vi "Solve_Special_PRB_101_Subtracks-2.vi"(3 "error IN":errorcluster, 5 "[IN] Subtracks":T1(array[cluster])) -> (0 "error OUT":errorcluster, 1 "[OUT] Special case!":bool, 2 "[OUT] Subtracks":T1(array[cluster]))   [LabVIEW 2013]
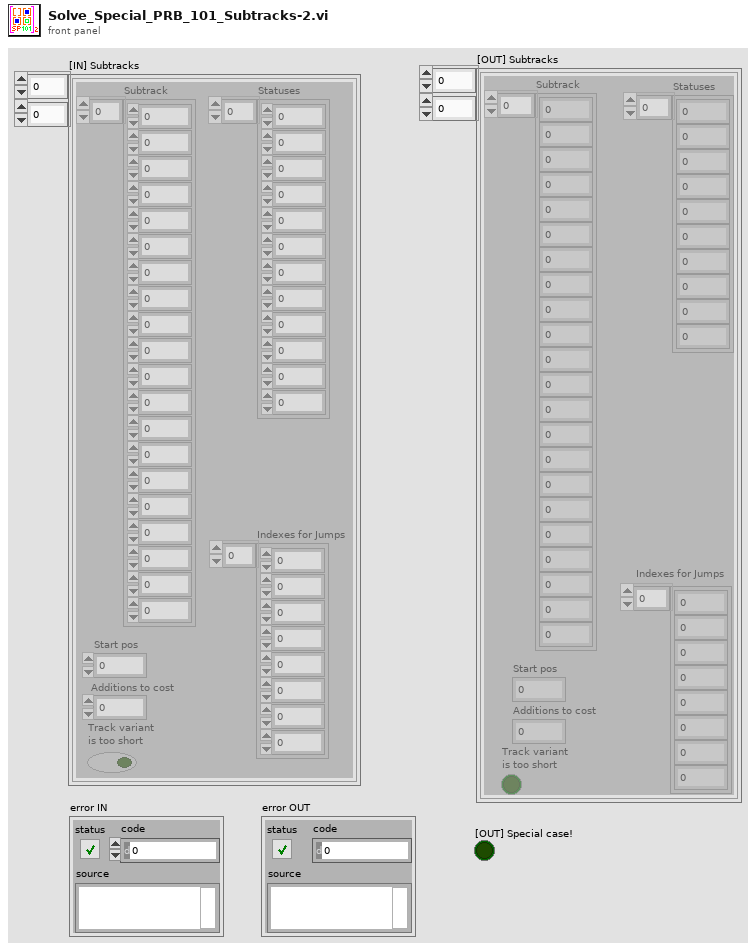
[diagram p1: front panel]
types:
  T1 = cluster{"Subtrack":dbl[], "Statuses":i16[], "Start pos":i32, "Additions to cost":i32, "Track variant \nis too short":bool, "Indexes for Jumps":i32[]}[][]
  T2 = cluster{"Subtrack":dbl[], "Statuses":i16[], "Start pos":i32, "Additions to cost":i32, "Track variant \nis too short":bool, "Indexes for Jumps":i32[]}
  T3 = cluster{"Subtrack":dbl[], "Statuses":i16[], "Start pos":i32, "Additions to cost":i32, "Track variant \nis too short":bool, "Indexes for Jumps":i32[]}[]
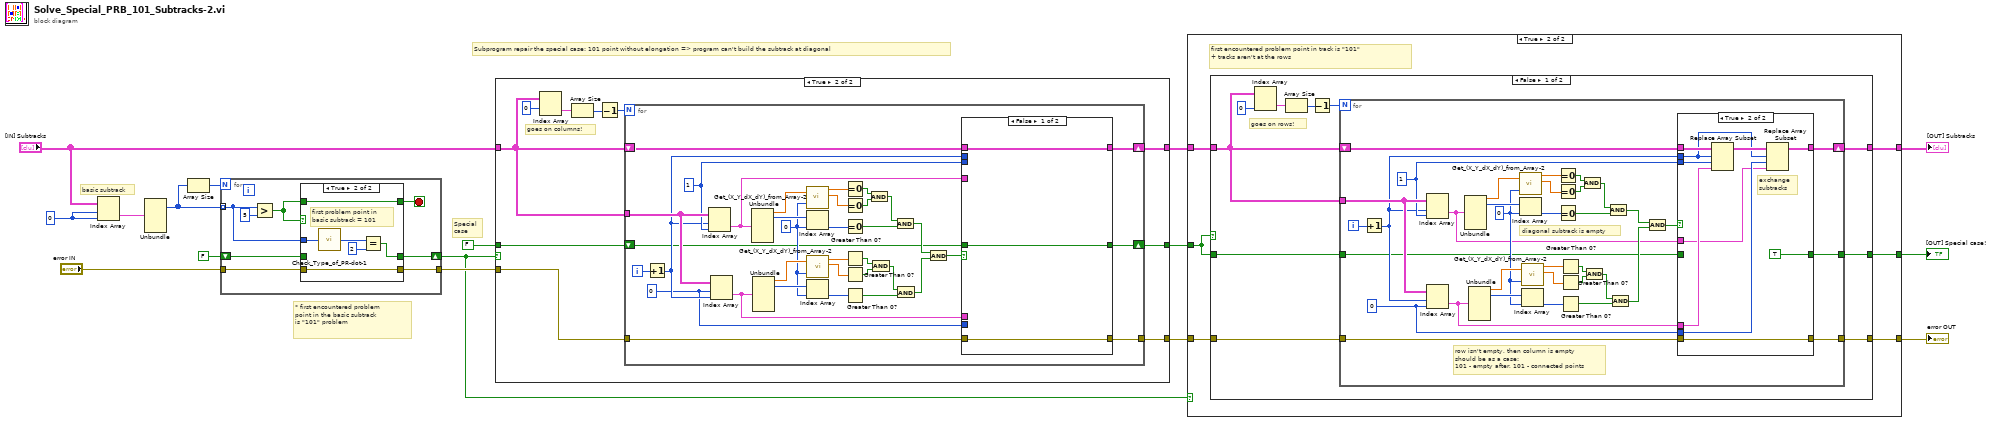
[diagram p0: block diagram]
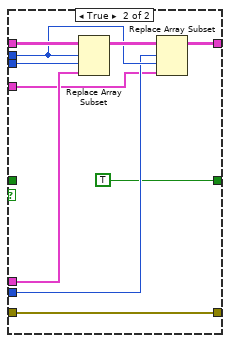
[diagram p6: hidden frame]
diagram:
  w16 = 0 ("index (row)")
  # "* first encountered problem\npoint in the basic subtrack\nis \"101\" problem"
  # "Special \ncase"
  # "Subprogram repair the special case: 101 point without elongation => program can't build the subtrack at diagonal"
  # "basic subtrack"
  n1 = Index Array(array="[IN] Subtracks", index (row)=w16, index (col)=w16) -> (element=w15:T2)
  n2 = Unbundle(w15) -> ("Statuses"=w13:i16[])  [unwired: 5 out]
  n3 = Array Size(array=w13) -> (size(s)=w14:i32)
  n4 = for {
    N: w14 -> [_]
    tunnel: w13 -> [w23] mode=indexing
    shift-right: [w19] -> w7
    shift-left: FALSE -> [w22]
    tunnel: "error IN" -> [w18]
    tunnel: [w17] -> w10
    stop <- w20 stop-if-true
    n5 = Greater?(x=w23, y=i16 5) -> (0:w21:bool)
    n6 = case shown="True" w21 {
      tunnel: w23 -> [_ w31]
      tunnel: w22 -> [w26 _]
      tunnel: w21 -> [w27 w30]
      tunnel: [w27 w30] -> w20
      tunnel: [w26 w29] -> w19
      tunnel: w18 -> [w25 w28]
      tunnel: [w25 w28] -> w17
      frame False {
      }
      frame True {
        # "first problem point in \nbasic subtrack = 101"
        n7 = call "Check_Type_of_PR-dot-1.vi"("[IN] dot status"=w31) -> ("[OUT] Type of\nproblem dot"=w33:i32)
        n8 = Equal?(x=w33, y=2) -> (x = y?=w29:bool)
      }
    }
  }
  n9 = case shown="True" w7 {
    tunnel: w10 -> [w35 w42]
    tunnel: "[IN] Subtracks" -> [w36 w45]
    tunnel: [w36 w40] -> w5
    tunnel: [w35 w41] -> w4
    tunnel: FALSE -> [w34 w39]
    tunnel: [w34 w38] -> w6
    frame False {
    }
    frame True {
      # "goes on columns!"
      n10 = Index Array(array=w45, index (row)=0 ("disabled index (col)")) -> (element=w46:T3)  [unwired: 1 in]
      n11 = Array Size(array=w46) -> (size(s)=w44:i32)
      n12 = Decrement(x=w44) -> (x-1=w43:i32)
      n13 = for {
        N: w43 -> [_]
        tunnel: w45 -> [w80]
        shift-right: [w51] -> w40
        shift-left: w45 -> [w57]
        tunnel: w42 -> [w50]
        tunnel: [w49] -> w41
        shift-right: [w47] -> w38
        shift-left: w39 -> [w48]
        i -> [w81]
        w65 = 0 ("index")
        w52 = 0 ("disabled index (col)")
        w54 = 1 ("disabled index (col)")
        n14 = Increment(x=w81) -> (x+1=w53:i32)
        n15 = Index Array(array=w80, index (row)=w53, index (col)=w54) -> (element=w56:T2)
        n16 = Index Array(array=w80, index (row)=w52, index (col)=w53) -> (element=w55:T2)
        n17 = Unbundle(w56) -> ("Subtrack"=w77:dbl[], "Statuses"=w79:i16[])  [unwired: 4 out]
        n18 = Unbundle(w55) -> ("Subtrack"=w76:dbl[], "Statuses"=w78:i16[])  [unwired: 4 out]
        n19 = call "Get_(X_Y_dX_dY)_from_Array-2.vi"("(X,Y,dX,dY)"=w77, "Index of Displacement"=w65) -> ("X"=w75:dbl, "Y"=w74:dbl)  [unwired: 2 out]
        n20 = Index Array(array=w79, index=w65) -> (element=w73:i16)
        n21 = call "Get_(X_Y_dX_dY)_from_Array-2.vi"("(X,Y,dX,dY)"=w76, "Index of Displacement"=w65) -> ("X"=w68:dbl, "Y"=w67:dbl)  [unwired: 2 out]
        n22 = Index Array(array=w78, index=w65) -> (element=w66:i16)
        n23 = Equal To 0?(x=w75) -> (x = 0?=w72:bool)
        n24 = Equal To 0?(x=w74) -> (x = 0?=w71:bool)
        n25 = Equal To 0?(x=w73) -> (x = 0?=w69:bool)
        n26 = Greater Than 0?(x=w68) -> (x > 0?=w64:bool)
        n27 = Greater Than 0?(x=w67) -> (x > 0?=w63:bool)
        n28 = Greater Than 0?(x=w66) -> (x > 0?=w61:bool)
        n29 = And(x=w72, y=w71) -> (x .and. y?=w70:bool)
        n30 = And(x=w64, y=w63) -> (x .and. y?=w62:bool)
        n31 = And(x=w70, y=w69) -> (x .and. y?=w60:bool)
        n32 = And(x=w62, y=w61) -> (x .and. y?=w59:bool)
        n33 = And(x=w60, y=w59) -> (x .and. y?=w58:bool)
        n34 = case shown="False" w58 {
          tunnel: w57 -> [w84 w94]
          tunnel: w56 -> [_ w88]
          tunnel: w55 -> [_ w92]
          tunnel: w53 -> [_ w90]
          tunnel: w54 -> [_ w93]
          tunnel: w52 -> [_ w89]
          tunnel: [w84 w87] -> w51
          tunnel: w50 -> [w83 w86]
          tunnel: [w83 w86] -> w49
          tunnel: w48 -> [w82 _]
          tunnel: [w82 TRUE] -> w47
          frame False {
          }
          frame True {
            n35 = Replace Array Subset(array=w94, new element=w92, index (row)=w90, index (col)=w93) -> (w91:T1)
            n36 = Replace Array Subset(array=w91, new element=w88, index (row)=w89, index (col)=w90) -> (w87:T1)
          }
        }
      }
    }
  }
  n37 = case shown="True" w7 {
    tunnel: w6 -> [w96 w101]
    tunnel: w5 -> [w95 w103]
    tunnel: w4 -> [w97 w102]
    tunnel: [w95 w100] -> w2
    tunnel: [w96 w99] -> w3
    tunnel: [w97 w98] -> w1
    frame False {
    }
    frame True {
      # "first encountered problem point in track is \"101\"\n+ tracks aren't at the rows"
      n38 = case shown="False" w101 {
        tunnel: w103 -> [w109 w164]
        tunnel: w102 -> [w107 w162]
        tunnel: w101 -> [w108 w163]
        tunnel: [w106 w164] -> w100
        tunnel: [w105 w163] -> w99
        tunnel: [w104 w162] -> w98
        frame False {
          # "goes on rows!"
          n39 = Index Array(array=w109, index (col)=0 ("index (row)")) -> (element=w112:T3)  [unwired: 1 in]
          n40 = Array Size(array=w112) -> (size(s)=w113:i32)
          n41 = Decrement(x=w113) -> (x-1=w111:i32)
          n42 = for {
            N: w111 -> [_]
            shift-right: [w117] -> w106
            shift-left: w109 -> [w124]
            tunnel: w109 -> [w138]
            tunnel: w108 -> [w116]
            tunnel: w107 -> [w122]
            tunnel: [w115] -> w105
            tunnel: [w114] -> w104
            i -> [w148]
            w119 = 0 ("disabled index (col)")
            w128 = 0 ("index")
            w121 = 1 ("disabled index (col)")
            # "row isn't empty, then column is empty\nshould be as a case:\n101 - empty after, 101 - connected points"
            # "diagonal subtrack is empty"
            n43 = Increment(x=w148) -> (x+1=w120:i32)
            n44 = Index Array(array=w138, index (row)=w120, index (col)=w121) -> (element=w118:T2)
            n45 = Index Array(array=w138, index (row)=w120, index (col)=w119) -> (element=w123:T2)
            n46 = Unbundle(w118) -> ("Subtrack"=w146:dbl[], "Statuses"=w147:i16[])  [unwired: 4 out]
            n47 = Unbundle(w123) -> ("Subtrack"=w136:dbl[], "Statuses"=w137:i16[])  [unwired: 4 out]
            n48 = call "Get_(X_Y_dX_dY)_from_Array-2.vi"("(X,Y,dX,dY)"=w146, "Index of Displacement"=w128) -> ("X"=w145:dbl, "Y"=w144:dbl)  [unwired: 2 out]
            n49 = Index Array(array=w147, index=w128) -> (element=w143:i16)
            n50 = call "Get_(X_Y_dX_dY)_from_Array-2.vi"("(X,Y,dX,dY)"=w136, "Index of Displacement"=w128) -> ("X"=w135:dbl, "Y"=w134:dbl)  [unwired: 2 out]
            n51 = Index Array(array=w137, index=w128) -> (element=w133:i16)
            n52 = Equal To 0?(x=w145) -> (x = 0?=w142:bool)
            n53 = Equal To 0?(x=w144) -> (x = 0?=w141:bool)
            n54 = Equal To 0?(x=w143) -> (x = 0?=w139:bool)
            n55 = Greater Than 0?(x=w135) -> (x > 0?=w132:bool)
            n56 = Greater Than 0?(x=w134) -> (x > 0?=w131:bool)
            n57 = Greater Than 0?(x=w133) -> (x > 0?=w129:bool)
            n58 = And(x=w142, y=w141) -> (x .and. y?=w140:bool)
            n59 = And(x=w132, y=w131) -> (x .and. y?=w130:bool)
            n60 = And(x=w140, y=w139) -> (x .and. y?=w127:bool)
            n61 = And(x=w130, y=w129) -> (x .and. y?=w126:bool)
            n62 = And(x=w127, y=w126) -> (x .and. y?=w125:bool)
            n63 = case shown="True" w125 {
              tunnel: w124 -> [w150 w161]
              tunnel: w123 -> [_ w159]
              tunnel: w122 -> [w151 w153]
              tunnel: w121 -> [_ w160]
              tunnel: w120 -> [_ w156]
              tunnel: w119 -> [_ w157]
              tunnel: w118 -> [_ w155]
              tunnel: [w150 w154] -> w117
              tunnel: [w151 w153] -> w114
              tunnel: w116 -> [w149 _]
              tunnel: [w149 TRUE] -> w115
              frame False {
              }
              frame True {
                # "exchange \nsubtracks"
                n64 = Replace Array Subset(array=w161, new element=w159, index (row)=w156, index (col)=w160) -> (w158:T1)
                n65 = Replace Array Subset(array=w158, new element=w155, index (row)=w156, index (col)=w157) -> (w154:T1)
              }
            }
          }
        }
        frame True {
        }
      }
    }
  }
  "error OUT" <- w1
  "[OUT] Subtracks" <- w2
  "[OUT] Special case!" <- w3
